vi "Calculate ref buffer dimensions.vi"(10 "Frames":i16, 11 "RefDAQParam in":T1={"Full Frame Size"=0, "Ref Field of View"=0.0, "Ref Zoom"=0, "Ref_dwellTime"=0.0, "Ref X-pixels-per-line(Npxr)"=0, "Ref Y-lines-per-image(Npyr)"=0, "Ref Z-lines-per-image"=0, "Ref Scan Cycles"=0, "Ref threshold"=0, "Ref average"=1, "Sliding Average"=FALSE, "proportioanl_scale"=1.5999755859375, "Integral_scale"=2047.9375, "proportioanl_scaleZ"=1.5999755859375, "Integral_scaleZ"=400.0, "Diff_threshold"=0.0, "Diff_threshold _z"=0.0, "scale"=0.0, "Control algorithm"=enum."Kalman", "New line trigger enabled"=TRUE, "Slide Averaging"=FALSE, "Ref count reset enabled"=FALSE} {"proportioanl_scaleZ" format="%#_15g"; "Diff_threshold" format="%#_15g"; "Diff_threshold _z" format="%#_15g"; "scale" format="%#_15g"; "proportioanl_scale" format="%#_15g"}) -> (1 "Ref Y-lines-per-image(Npyr)":i16, 2 "Ref X-pixels-per-line(Npxr)":i16, 3 "Y lines  + Z lines":i16, 4 "Ref Z-lines-per-image":i16, 5 "Number of pixels per frame":i16, 7 "Total number of pixels":i16)   [LabVIEW 2017]
uses:
  Typedefs/Ref DAQ Param.ctl
  Movement Correction/Typedefs/Control algorithm.ctl
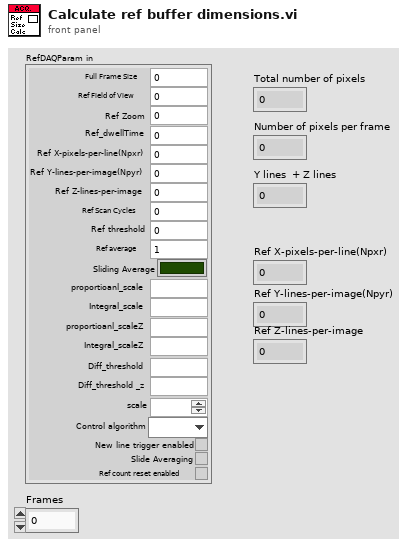
[diagram p1: front panel]
types:
  T1 = typedef "Ref DAQ Param.ctl" = cluster{"Full Frame Size":u16, "Ref Field of View":sgl, "Ref Zoom":i8, "Ref_dwellTime":sgl, "Ref X-pixels-per-line(Npxr)":i16, "Ref Y-lines-per-image(Npyr)":i16, "Ref Z-lines-per-image":i16, "Ref Scan Cycles":i32, "Ref threshold":u16, "Ref average":u16, "Sliding Average":bool, "proportioanl_scale":fxp<+,16,2>, "Integral_scale":fxp<+/-,16,12>, "proportioanl_scaleZ":fxp<+,16,2>, "Integral_scaleZ":fxp<+/-,16,12>, "Diff_threshold":fxp<+,16,2>, "Diff_threshold _z":fxp<+,16,2>, "scale":fxp<+,16,2>, "Control algorithm":T2, "New line trigger enabled":bool, "Slide Averaging":bool, "Ref count reset enabled":bool}
  T2 = typedef "Control algorithm.ctl" = enum16{"PID", "Kalman"}
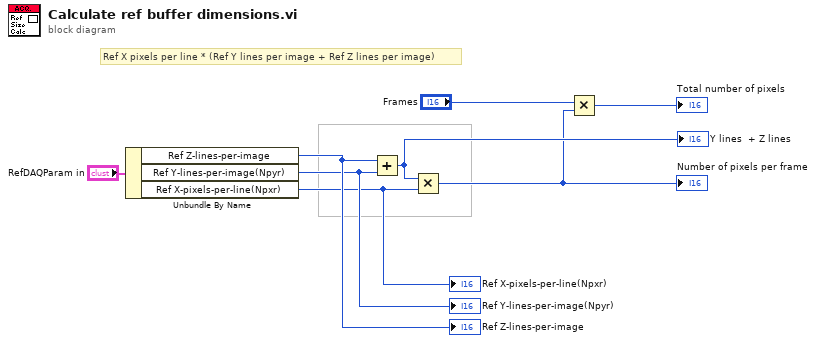
[diagram p0: block diagram]
diagram:
  # "Ref X pixels per line * (Ref Y lines per image + Ref Z lines per image)"
  n1 = Unbundle By Name("RefDAQParam in") -> ("Ref Z-lines-per-image"=w7:i16, "Ref Y-lines-per-image(Npyr)"=w6:i16, "Ref X-pixels-per-line(Npxr)"=w4:i16)
  "Ref X-pixels-per-line(Npxr)" <- w4
  "Ref Y-lines-per-image(Npyr)" <- w6
  "Ref Z-lines-per-image" <- w7
  n2 = Add(x=w7, y=w6) -> (x+y=w5:i16)
  "Y lines  + Z lines" <- w5
  n3 = Multiply(x=w5, y=w4) -> (x*y=w3:i16)
  "Number of pixels per frame" <- w3
  n4 = Multiply(x="Frames", y=w3) -> (x*y=→"Total number of pixels":i16)
